vi "pr2c.vi"() -> ()   [LabVIEW 2013]
uses:
  <vilib>/Platform/TimedLoop/XDataNode/timing_clust.ctl
  <vilib>/Platform/TimedLoop/XDataNode/nitl_modes.ctl
  <vilib>/Platform/TimedLoop/XDataNode/wakeup.ctl
  <vilib>/DAQmx/write.llb/DAQmx Write (Counter Frequency 1Chan 1Samp).vi
  <vilib>/DAQmx/read.llb/DAQmx Read (Counter DBL 1Chan 1Samp).vi
  <vilib>/DAQmx/write.llb/DAQmx Write (Digital Bool 1Line 1Point).vi
  <vilib>/DAQmx/create/channels.llb/DAQmx Create Channel (CI-Position-Angular Encoder).vi
  <vilib>/DAQmx/create/channels.llb/DAQmx Create Channel (DO-Digital Output).vi
  <vilib>/DAQmx/create/channels.llb/DAQmx Create Channel (CO-Pulse Generation-Frequency).vi
  <vilib>/DAQmx/configure/timing.llb/DAQmx Timing (Implicit).vi
  <vilib>/Utility/file.llb/Write To Spreadsheet File (DBL).vi
  <vilib>/DAQmx/miscellaneous.llb/DAQmx Fill In Error Info.vi
  <vilib>/platform/TimedLoop/XDataNode/XDataNode.xnode
  <vilib>/Platform/TimedLoop/XDataNode/XDNodeRunTimeDep.lvlib
panel:
  in  "Señal a generar":enum16{"Chirp", "Archivo", "Step", "PRBS"}(ring)=enum."Archivo"
  out "ticks por Tm":dbl
  out "Salida":waveform(dbl)(graph)
  out "size(s)":i32
  out "offset":dbl
  in  "Rango Frec para chrip":cluster{"start freq":dbl, "end freq":dbl}={"start freq"=0.5, "end freq"=2.0} {"end freq" format="%0.2f"; "start freq" format="%0.2f"}
  in  "Puntos a generar-chirp":i32=100
  in  "amplitude":dbl=0.1 format="%0.2f"
  in  "Zona muerta":dbl=0.2
  out "Señales Normalizadas":waveform(dbl)[](graph)
  in  "Numero de ciclos de \nPWM por periodo de muestreo (N)":dbl=20.0
  in  "Counter (s)":tag="Dev1/ctr0"
  in  "Periodo de muestreo (seg)":dbl=0.05
  out "Entrada":waveform(dbl)(graph)
  out "Error":errorcluster
  in  "Salida para DIR":tag="Dev1/port0/line0"
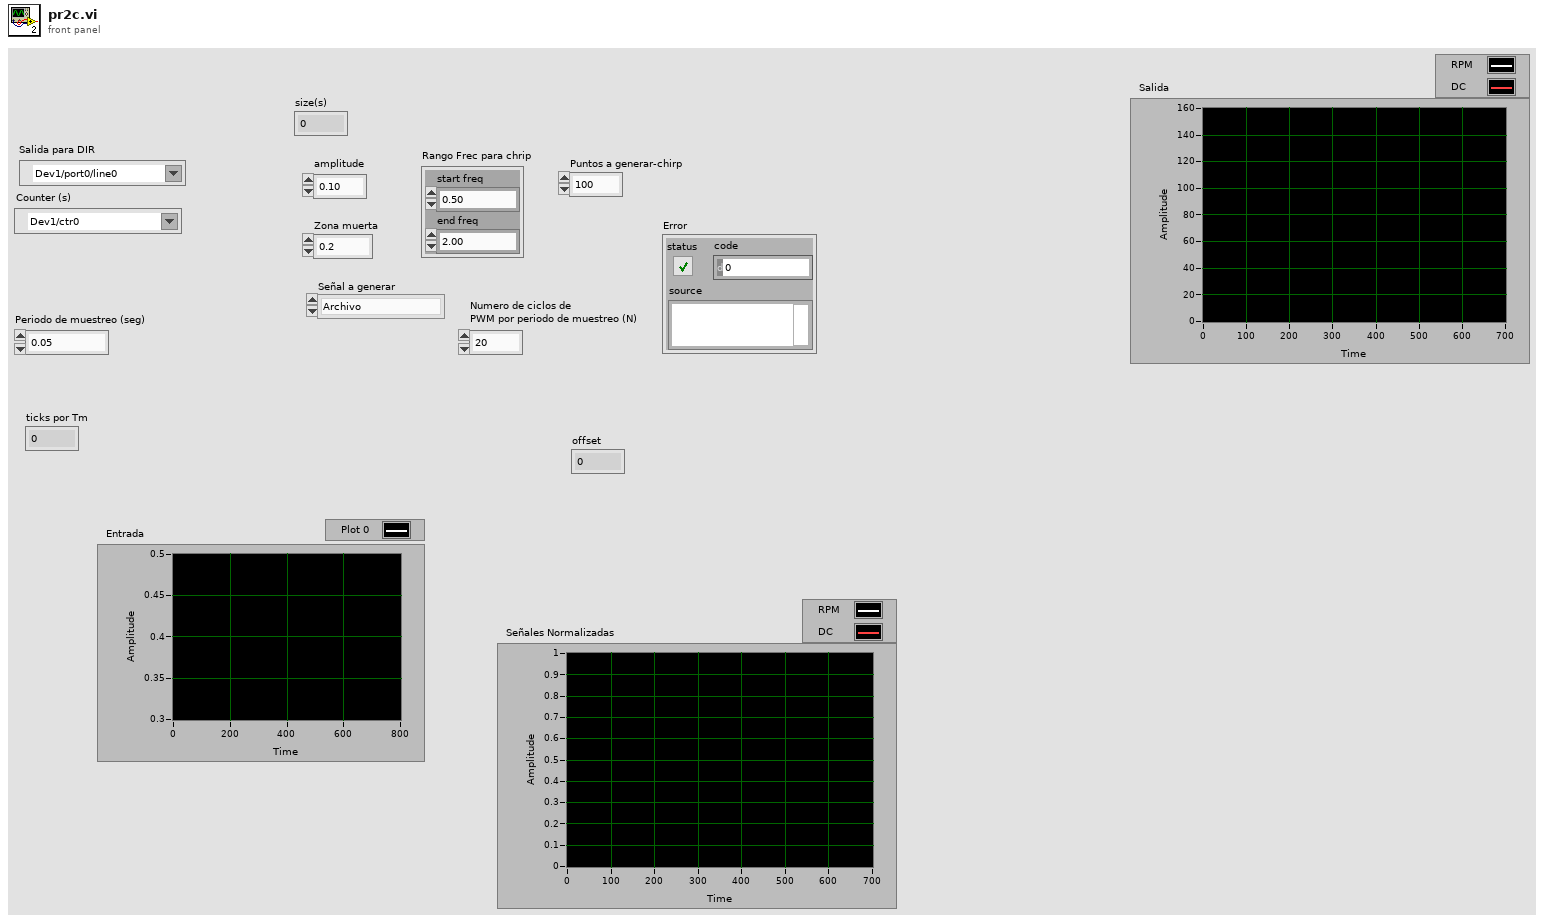
[diagram p1: front panel]
types:
  T1 = typedef "XDNodeRunTimeDep.lvlib/timing_clust.ctl" = cluster{"Expected End [f-1]":u64, "Actual End [f-1]":u64, "Finished Late? [f-1]":bool, "Expected End [i-1]":u64, "Actual End [i-1]":u64, "Finished Late? [i-1]":bool, "Expected Start [i]":u64, "Actual Start [i]":u64, "Expected Start [f]":u64, "Actual Start [f]":u64, "Source Name":string, "Structure Name":string, "Period":i64, "Deadline":i64, "Offset":i64, "Start":i64, "Priority":i32, "Timeout":i32, "Mode":T2, "Wakeup Reason":T3, "Error":errorcluster, "Source Type":string, "Secondary Source Type":string, "Global End Time":u64, "Global Start Time":u64, "Frame Duration":u64, "Iteration Duration":u64, "Assigned CPU":i32, "I/O Scan Engine Mode":u32}
  T2 = typedef "XDNodeRunTimeDep.lvlib/nitl_modes.ctl" = enum32{"No Change", "Process missed periods, maintain original phase", "Discard missed periods, maintain original phase", "Process missed periods, ignore original phase", "Discard missed periods, ignore original phase"}
  T3 = typedef "XDNodeRunTimeDep.lvlib/wakeup.ctl" = enum32{"Normal", "Aborted", "Asynchronous wakeup", "Timing source error", "Timed loop error", "Timeout"}
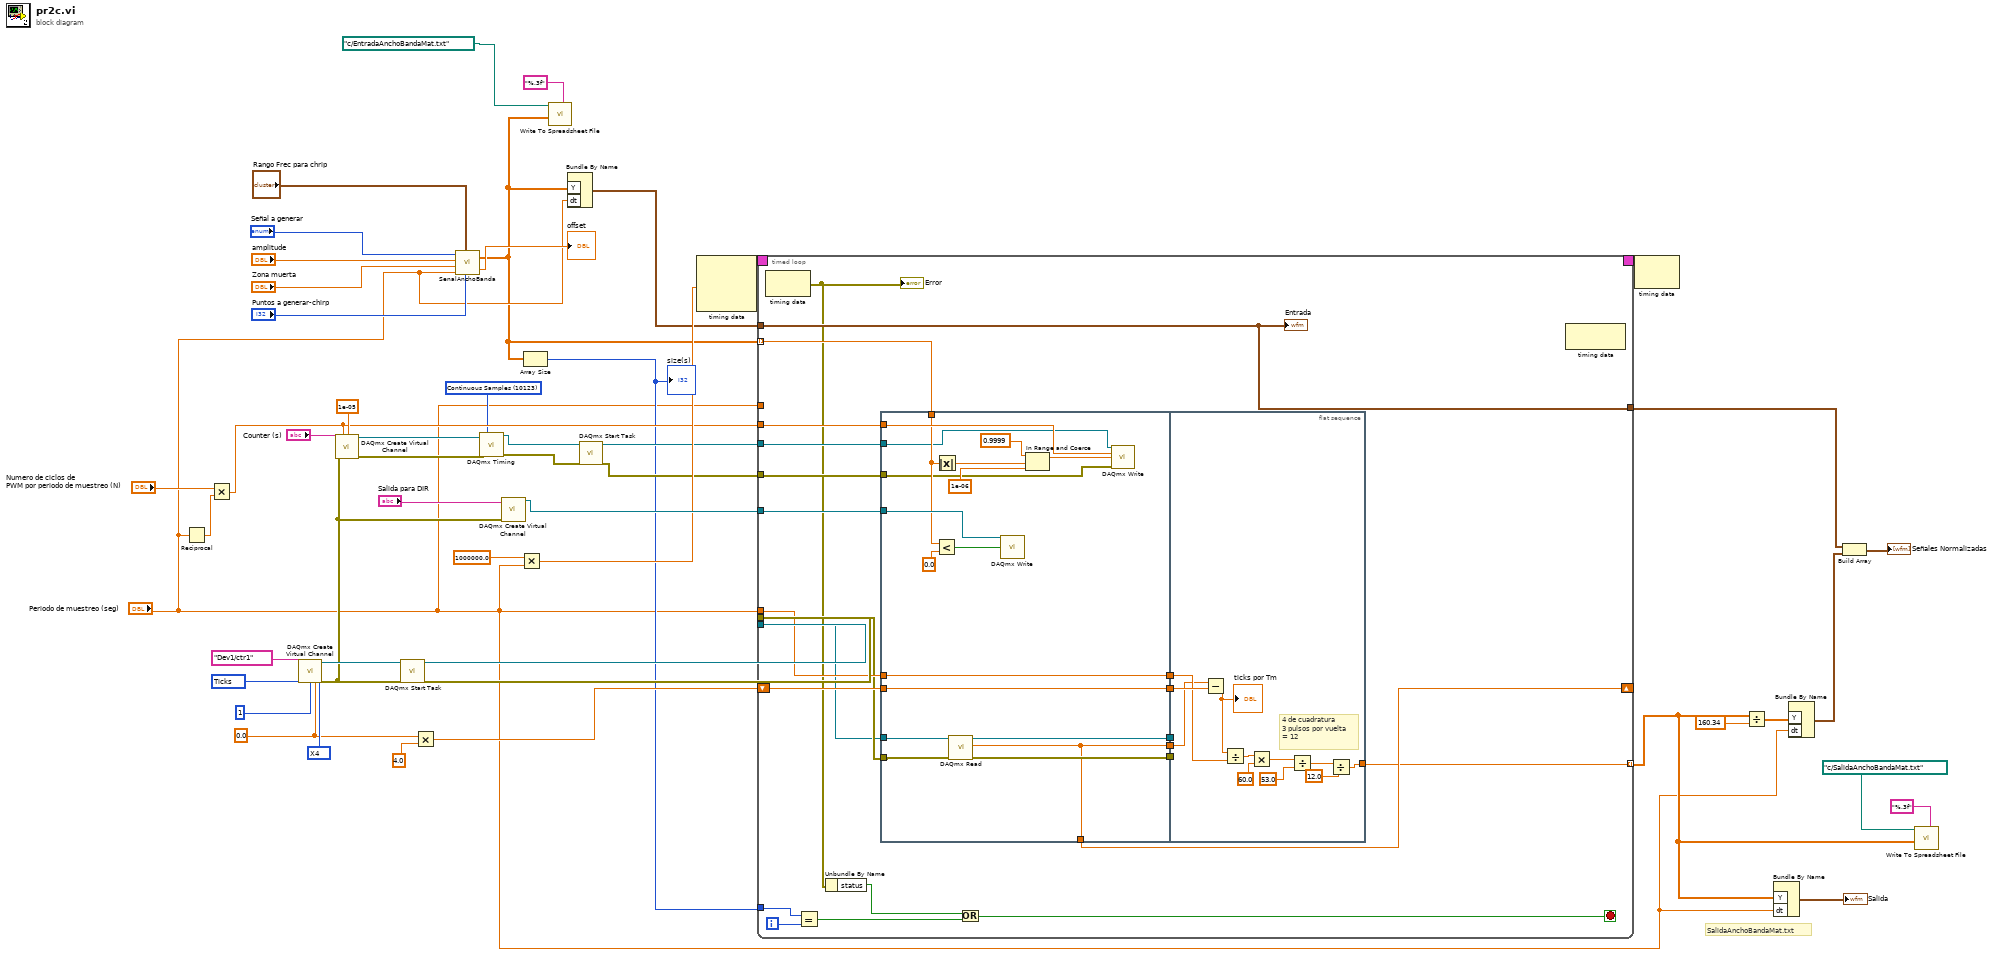
[diagram p0: block diagram]
diagram:
  w22 = 10123 items=["Finite Samples"=10178, "Continuous Samples"=10123, "Hardware Timed Single Point"=12522] ("sample mode")
  w45 = 10092 items=["X1"=10090, "X2"=10091, "X4"=10092, "Two Pulse Counting"=10313] ("decoding type")
  w40 = 0.0 ("initial angle")
  w47 = 10304 items=["Degrees"=10146, "Radians"=10273, "Ticks"=10304, "From Custom Scale"=10065] ("units")
  # "SalidaAnchoBandaMat.txt"
  n1 = Reciprocal(x="Periodo de muestreo (seg)") -> (1/x=w29:dbl)
  n2 = Multiply(x="Numero de ciclos de \nPWM por periodo de muestreo (N)", y=w29) -> (x*y=w30:dbl)
  n3 = call-poly <vilib>:"DAQmx Create Virtual Channel.vi"("counter"=tag "Dev1/ctr1", "decoding type"=w45, "units"=w47, "pulses per revolution"=u32 1, "initial angle"=w40) -> ("task out"=w44:refnum<k21>, "error out"=w32:errorcluster)  [unwired: 9 in]
  n4 = call-poly <vilib>:"DAQmx Create Virtual Channel.vi"("frequency"=w30, "duty cycle"=1e-05, "counter"="Counter (s)", "error in"=w32) -> ("task out"=w28:refnum<k21>, "error out"=w25:errorcluster)  [unwired: 10 in]
  n5 = call <vilib>:"DAQmx Start Task.vi"("task/channels in"=w44, "error in"=w32) -> ("task out"=w43:refnum<k21>, "error out"=w42:errorcluster)  [unwired: 12 in]
  n6 = Multiply(x=w40, y=4.0) -> (x*y=w31:dbl)
  n7 = call "SenalAnchoBanda.vi"("Puntos a generar-chirp"="Puntos a generar-chirp", "Rango Frec para chrip"="Rango Frec para chrip", "Tm"="Periodo de muestreo (seg)", "Zona muerta"="Zona muerta", "amplitude"="amplitude", "Señal a generar"="Señal a generar") -> ("offset"=→"offset":dbl, "Señal"=w3:dbl[])
  n8 = call-poly <vilib>:"DAQmx Timing.vi"("task/channels in"=w28, "sample mode"=w22, "error in"=w25) -> ("task out"=w27:refnum<k21>, "error out"=w24:errorcluster)  [unwired: 11 in]
  n9 = call-poly <vilib>:"DAQmx Create Virtual Channel.vi"("lines"="Salida para DIR", "error in"=w32) -> ("task out"=w37:refnum<k21>)  [unwired: 12 in, 1 out]
  n10 = Multiply(x=1000000.0, y="Periodo de muestreo (seg)") -> (x*y=w36:dbl)
  n11 = Array Size(array=w3) -> (size(s)=w11:i32)
  "size(s)" <- w11
  n12 = call-poly <vilib>:"Write To Spreadsheet File.vi"("format (%.3f)"="%.3f", "1D data"=w3, "file path (dialog if empty)"=path "c:/EntradaAnchoBandaMat.txt") -> ()  [unwired: 5 in, 1 out]
  n13 = Bundle By Name("Y"=w3, "dt"="Periodo de muestreo (seg)") -> (w12:waveform(dbl))  [unwired: 1 in]
  n14 = call <vilib>:"DAQmx Start Task.vi"("task/channels in"=w27, "error in"=w24) -> ("task out"=w26:refnum<k21>, "error out"=w23:errorcluster)  [unwired: 12 in]
  n15 = node-c288(w36) -> (w50:T1)  [unwired: 2 in]
  n16 = timed-loop {
    timing: w50 -> [_]
    timing-out: [_] -> w49
    shift-right: [w64] -> _
    shift-left: w31 -> [w73]
    tunnel: w43 -> [w66]
    tunnel: w42 -> [w67]
    tunnel: "Periodo de muestreo (seg)" -> [w72]
    tunnel: w3 -> [w60] mode=indexing
    tunnel: "Periodo de muestreo (seg)" -> [_]
    tunnel: w37 -> [w69]
    tunnel: w12 -> [w57]
    tunnel: w30 -> [w61]
    tunnel: w26 -> [w59]
    tunnel: w23 -> [w58]
    tunnel: [w55] -> w7 mode=indexing
    tunnel: [w57] -> w21
    tunnel: w11 -> [w56]
    i -> [w62]
    stop <- w51 stop-if-true
    n17 = node-c288() -> (w54:errorcluster)  [unwired: 1 in]
    "Error" <- w54
    n18 = Equal?(x=w56, y=w62) -> (x = y?=w53:bool)
    n19 = Unbundle By Name(w54) -> ("status"=w52:bool)
    n20 = flat-sequence {
      tunnel: w72 -> [w90]
      tunnel: w73 -> [w91]
      tunnel: [w91] -> w71
      tunnel: [w90] -> w70
      tunnel: w69 -> [w85]
      tunnel: [w82] -> w68
      tunnel: w67 -> [w81]
      tunnel: w66 -> [w80]
      tunnel: [w79] -> w65
      tunnel: [w78] -> w64
      tunnel: [w78] -> w63
      tunnel: w61 -> [w77]
      tunnel: w60 -> [w76]
      tunnel: w59 -> [w75]
      tunnel: w58 -> [w74]
      tunnel: [w93] -> w55
      tunnel: w71 -> [w102]
      tunnel: w70 -> [w96]
      tunnel: w68 -> [_]
      tunnel: w65 -> [_]
      tunnel: w63 -> [w95]
      frame #0 {
        n21 = Less?(x=w76, y=0.0) -> (x < y?=w83:bool)
        n22 = Absolute Value(x=w76) -> (abs(x)=w87:dbl)
        n23 = call-poly <vilib>:"DAQmx Read.vi"("task/channels in"=w80, "error in"=w81) -> ("task out"=w79:refnum<k21>, "data"=w78:dbl, "error out"=w82:errorcluster)  [unwired: 11 in]
        n24 = call-poly <vilib>:"DAQmx Write.vi"("task/channels in"=w85, "data"=w83) -> ()  [unwired: 11 in, 3 out]
        n25 = In Range and Coerce(upper limit=0.9999, x=w87, lower limit=1e-06) -> (coerced(x)=w86:dbl)  [unwired: 1 out]
        n26 = call-poly <vilib>:"DAQmx Write.vi"("task/channels in"=w75, "frequency"=w77, "duty cycle"=w86, "error in"=w74) -> ()  [unwired: 9 in, 3 out]
      }
      frame #1 {
        # "4 de cuadratura\n3 pulsos por vuelta\n= 12"
        n27 = Subtract(x=w95, y=w102) -> (x-y=w101:dbl)
        "ticks por Tm" <- w101
        n28 = Divide(x=w101, y=w96) -> (x/y=w100:dbl)
        n29 = Multiply(x=w100, y=60.0) -> (x*y=w98:dbl)
        n30 = Divide(x=w98, y=53.0) -> (x/y=w94:dbl)
        n31 = Divide(x=w94, y=12.0) -> (x/y=w93:dbl)
      }
    }
    n32 = Or(x=w52, y=w53) -> (x .or. y?=w51:bool)
    n33 = node-c288() -> ()  [unwired: 1 in, 1 out]
    "Entrada" <- w57
  }
  n34 = node-c288(w49) -> ()  [unwired: 1 out]
  n35 = Divide(x=w7, y=160.34) -> (x/y=w19:dbl[])
  n36 = Bundle By Name("Y"=w7, "dt"="Periodo de muestreo (seg)") -> (→"Salida":waveform(dbl))  [unwired: 1 in]
  n37 = Bundle By Name("Y"=w19, "dt"="Periodo de muestreo (seg)") -> (w18:waveform(dbl))  [unwired: 1 in]
  n38 = Build Array(w21, w18) -> (→"Señales Normalizadas":waveform(dbl)[])
  n39 = call-poly <vilib>:"Write To Spreadsheet File.vi"("format (%.3f)"="%.3f", "1D data"=w7, "file path (dialog if empty)"=path "c:/SalidaAnchoBandaMat.txt") -> ()  [unwired: 5 in, 1 out]
